vi "finalize initialization.vi"(8 "error in":errorcluster, 10 "configuration in":refnum<class "fixed channel configuration.lvclass">, 11 "fixed channel runtime in":refnum<class "fixed channel runtime.lvclass">) -> (0 "error out":errorcluster, 3 "fixed channel runtime out":refnum<class "fixed channel runtime.lvclass">)   [LabVIEW 2013, in "fixed channel runtime.lvclass"]
uses:
  fixed channel runtime.lvclass
  configuration/fixed channel configuration.lvclass
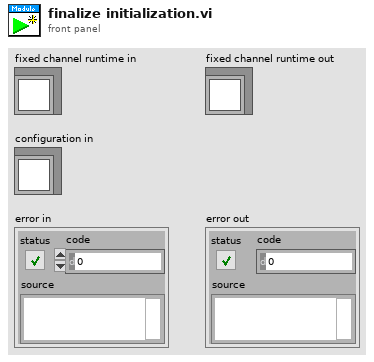
[diagram p1: front panel]
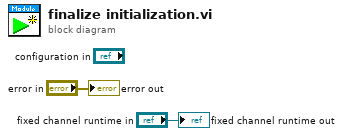
[diagram p0: block diagram]
diagram:
  "error out" <- "error in"
  "fixed channel runtime out" <- "fixed channel runtime in"
